vi "sub_str.vi"() -> ()   [LabVIEW 2019]
uses:
  <vilib>/RTI DDS Toolkit/Types/RTI DDS Advanced Writer Configuration.ctl
  <vilib>/RTI DDS Toolkit/VIs/AdvancedCreateWriter_String.vi
  <vilib>/RTI DDS Toolkit/VIs/Read_String.vi
  <vilib>/RTI DDS Toolkit/Library/LVDDS_library.lvlib
panel:
  out "error out":errorcluster
  out "Data":string
  in  "stop":bool
  in  "Topic Name":string="rt/mystrtopic"
  in  "Domain Id":u32
  in  "Advanced Writer Configuration":T1={"typeName"="std_msgs::msg::dds_::String_", "keyName"="", "domainParticipantQoSProfile"="", "dataWriterQoSProfile"="", "forceArrayMapping?"=FALSE, "forceUnboundedString?"=FALSE}
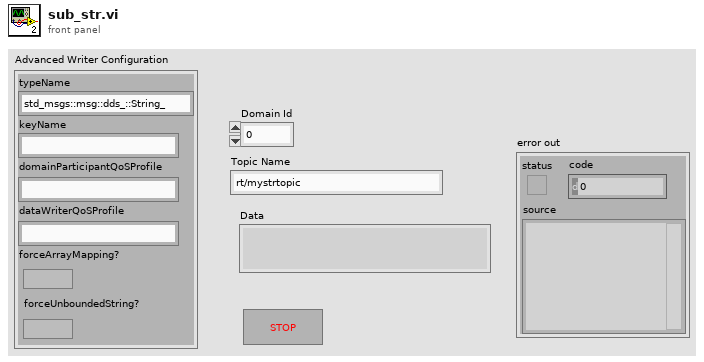
[diagram p1: front panel]
types:
  T1 = typedef "LVDDS_library.lvlib/RTI DDS Advanced Writer Configuration.ctl" = cluster{"typeName":string, "keyName":string, "domainParticipantQoSProfile":string, "dataWriterQoSProfile":string, "forceArrayMapping?":bool, "forceUnboundedString?":bool}
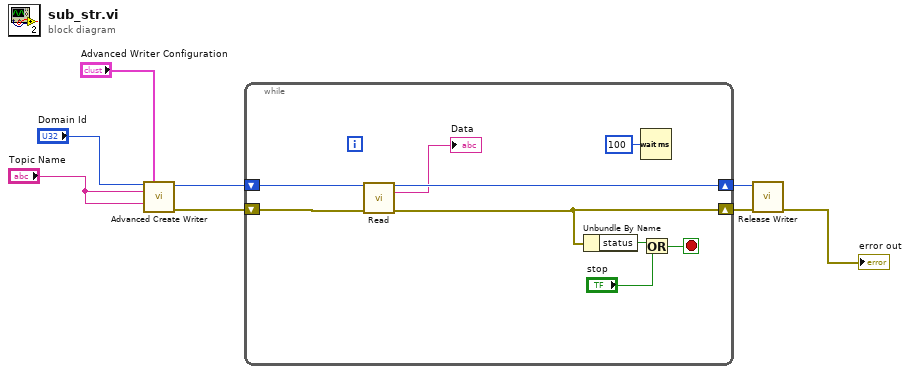
[diagram p0: block diagram]
diagram:
  n1 = call-poly <vilib>:"Advanced Create Writer.vi"("Domain Id"="Domain Id", "Advanced Writer Configuration"="Advanced Writer Configuration", "Topic Name"="Topic Name", "Data Type"="Topic Name") -> ("DDS Object Ref"=w5:u64, "error out"=w8:errorcluster)  [unwired: 10 in]
  n2 = while {
    shift-right: [w14] -> w7
    shift-left: w8 -> [w17]
    shift-right: [w16] -> w6
    shift-left: w5 -> [w15]
    stop <- w12 stop-if-true
    n3 = call-poly <vilib>:"Read.vi"("DDS Object Ref in"=w15, "error in (no error)"=w17) -> ("DDS Object Ref out"=w16:u64, "Data"=→"Data":string, "error out"=w14:errorcluster)  [unwired: 9 in, 2 out]
    n4 = Unbundle By Name(w14) -> ("status"=w13:bool)
    n5 = Wait (ms)(milliseconds to wait=u32 100) -> ()  [unwired: 1 out]
    n6 = Or(x=w13, y="stop") -> (x .or. y?=w12:bool)
  }
  n7 = call <vilib>:"Release Writer.vi"("error in (no error)"=w7, "DDS Object Ref"=w6) -> ("error out"=→"error out":errorcluster)  [unwired: 9 in]
